vi "rethinkdb_initialize_handshake.vi"(8 "error in (no error)":errorcluster, 10 "version (10=v1_0)":u8=10, 11 "rethinkdb in":refnum<k5>) -> (0 "error out":errorcluster, 2 "handshake":T1, 3 "rethinkdb out":refnum<k5>)   [LabVIEW 2017]
uses:
  f44fec32-2c35-428b-bc14-1cc76f2dec70.vi
  tcp/rethinkdb_tcp_write.vi
  tcp/rethinkdb_tcp_read.vi
  tcp/rethinkdb_tcp_parse_messages.vi
  tcp/rethinkdb_tcp_parse_errors.vi
  json/rethinkdb_json_load.vi
panel:
  in  "timeout ms (10000)":i32=10000
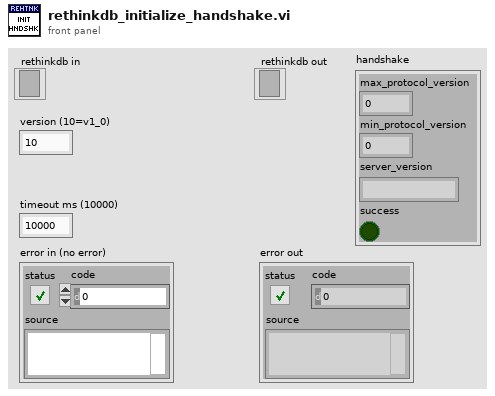
[diagram p1: front panel]
types:
  T1 = cluster{"max_protocol_version":u64, "min_protocol_version":u64, "server_version":string, "success":bool}
  T2 = enum16{"big-endian, network order", "native, host order", "little-endian"}
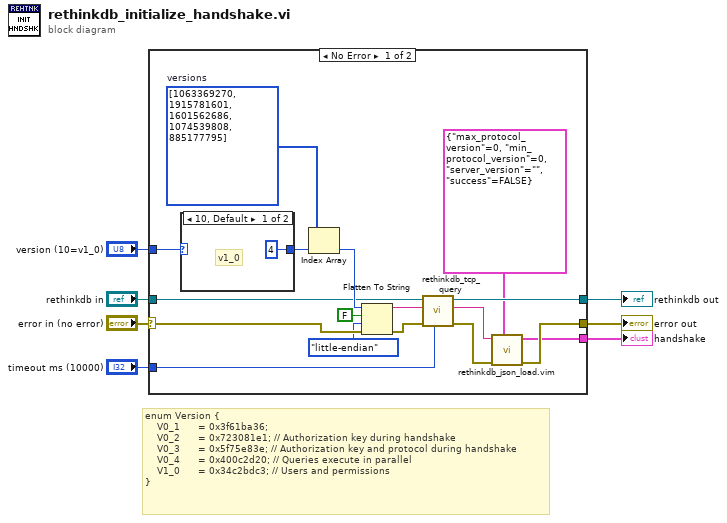
[diagram p0: block diagram]
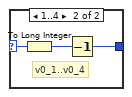
[diagram p2: hidden frame]
diagram:
  # "enum Version {\n    V0_1      = 0x3f61ba36;\n    V0_2      = 0x723081e1; // Authorization key during handshake\n    V0_3      = 0x5f75e83e; // Authorization key and protocol during handshake\n    V0_4      = 0x400c2d20; // Queries execute in parallel\n    V1_0      = 0x34c2bdc3; // Users and permissions\n}"
  n1 = case shown="No Error" "error in (no error)" {
    selector: "error in (no error)" -> [w21 w30]
    tunnel: "version (10=v1_0)" -> [w24 _]
    tunnel: [w10 w30] -> w5
    tunnel: "rethinkdb in" -> [w15 w29]
    tunnel: [w14 w29] -> w3
    tunnel: "timeout ms (10000)" -> [w13 _]
    tunnel: [w8 _] -> w1
    frame No Error {
      w22 = u32[] [1063369270, 1915781601, 1601562686, 1074539808, 885177795]  # versions
      n2 = case shown="10, Default" w24 {
        selector: w24 -> [_ w28]
        tunnel: [4 w26] -> w23
        frame 10, Default {
          # "v1_0"
        }
        frame 1..4 {
          # "v0_1..v0_4"
          n3 = To Long Integer(number=w28) -> (32bit integer=w27:i32)
          n4 = Decrement(x=w27) -> (x-1=w26:i32)
        }
      }
      n5 = Index Array(array=w22, index=w23) -> (element=w20:u32)
      n6 = Flatten To String(anything=w20, prepend array or string size? (T)=FALSE, byte order (0:big-endian, network order)=T2."little-endian", error in (no error)=w21) -> (data string=w16:string, error out=w17:errorcluster)  [unwired: 1 out]
      n7 = call "rethinkdb_tcp_query.vi"("timeout ms (10000)"=w13, "error in (no error)"=w17, "data in"=w16, "rethinkdb in"=w15) -> ("error out"=w11:errorcluster, "first message"=w12:string, "rethinkdb out"=w14:refnum<k5>)  [unwired: 4 in, 1 out]
      n8 = call "rethinkdb_json_load.vim"("type"=T1 {"max_protocol_version"=0, "min_protocol_version"=0, "server_version"="", "success"=FALSE} ("handshake"), "error in (no error)"=w11, "json"=w12) -> ("error out"=w10:errorcluster, "data out"=w8:T1)  [unwired: 7 in]
    }
    frame Error {
    }
  }
  "error out" <- w5
  "rethinkdb out" <- w3
  "handshake" <- w1
